vi "Untitled 1.vi"() -> ()   [LabVIEW 2014]
panel:
  out "initialized array":i32[][](array[numeric])
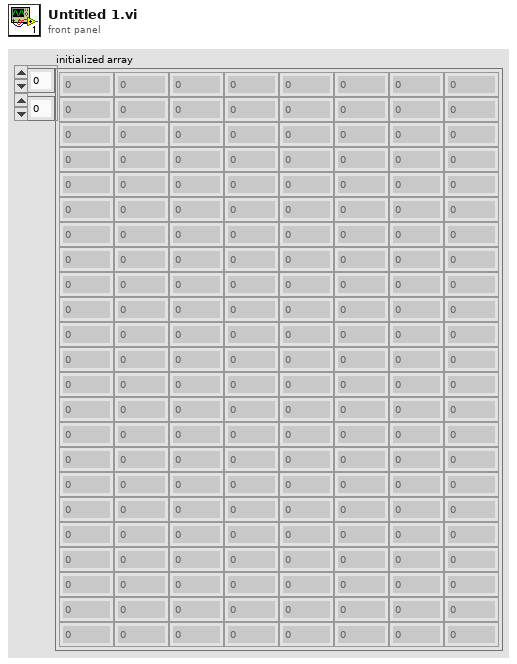
[diagram p1: front panel]
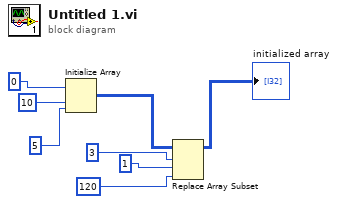
[diagram p0: block diagram]
diagram:
  n1 = Initialize Array(0, 10, 5) -> (w5:i32[][])
  n2 = Replace Array Subset(array=w5, new element=120, index (row)=3, index (col)=1) -> (→"initialized array":i32[][])
